vi "GetFullscreenDisplayModes.vi"(8 "No Error":errorcluster, 11 "DisplayID":T2) -> (0 "Error Out":errorcluster, 3 "Display Modes":T1[](array[typedef]))   [LabVIEW 2024, in "SDL3.lvlib" / "Video.lvlib"]
doc: "<B>Summary</B>\nGet a list of fullscreen display modes available on a display.\n\n<B>Remarks</B>\nThe display modes are sorted in this priority:\n\nw -> largest to smallest\nh -> largest to smallest\nbits per pixel -> more colors to fewer colors\npacked pixel layout -> largest to smallest\nrefresh rate -> highest to lowest\npixel density -> lowest to highest"
uses:
  Video.lvlib
  DisplayID--integer.ctl
  DisplayMode--cluster.ctl
  Pixels/PixelFormat--enum.ctl
  Dereference-DisplayMode.vi/d7f35e20-2a2c-4e03-b91a-a2fa7be3e3c2.vi
  Dereference-DisplayMode.vi/9072d7ce-49ca-4829-bd8f-b245b58a6c9d.vi
  Pixels/U32ToPixelFormatEnum.vi
  <vilib>/Utility/error.llb/Error Cluster From Error Code.vi
  Error/Error.lvlib
  Lib/SDL3-32.dll
  Stdinc/Stdinc.lvlib
  LV-Utilities/LV-Utilities.lvlib
  Pixels/Pixels.lvlib
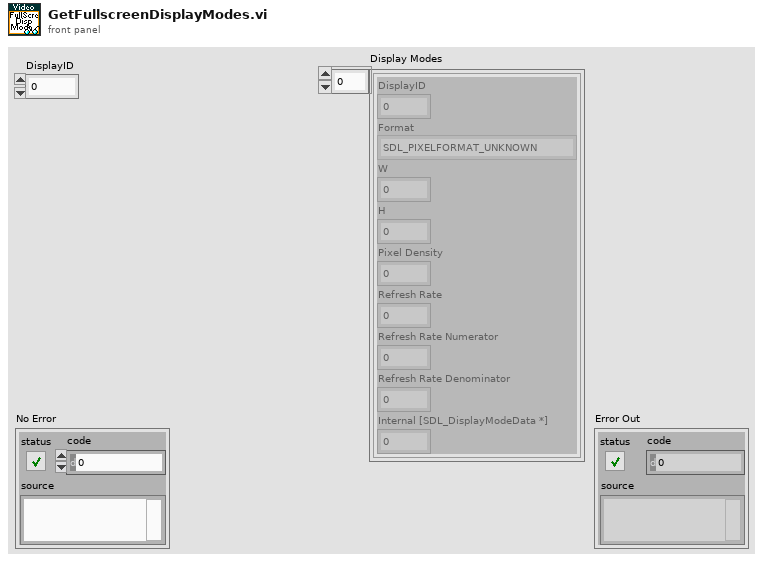
[diagram p1: front panel]
types:
  T1 = typedef "SDL3.lvlib/Video.lvlib/DisplayMode--cluster.ctl" = cluster{"DisplayID":T2, "Format":T3, "W":i32, "H":i32, "Pixel Density":sgl, "Refresh Rate":sgl, "Refresh Rate Numerator":i32, "Refresh Rate Denominator":i32, "Internal [SDL_DisplayModeData *]":i64}
  T2 = typedef "SDL3.lvlib/Video.lvlib/DisplayID--integer.ctl" = u32
  T3 = typedef "SDL3.lvlib/Pixels.lvlib/PixelFormat--enum.ctl" = enum32{"SDL_PIXELFORMAT_UNKNOWN", "SDL_PIXELFORMAT_INDEX1LSB", "SDL_PIXELFORMAT_INDEX1MSB", "SDL_PIXELFORMAT_INDEX2LSB", "SDL_PIXELFORMAT_INDEX2MSB", "SDL_PIXELFORMAT_INDEX4LSB", "SDL_PIXELFORMAT_INDEX4MSB", "SDL_PIXELFORMAT_INDEX8", "SDL_PIXELFORMAT_RGB332", "SDL_PIXELFORMAT_XRGB4444", "SDL_PIXELFORMAT_XBGR4444", "SDL_PIXELFORMAT_XRGB1555", "SDL_PIXELFORMAT_XBGR1555", "SDL_PIXELFORMAT_ARGB4444", "SDL_PIXELFORMAT_RGBA4444", "SDL_PIXELFORMAT_ABGR4444", "SDL_PIXELFORMAT_BGRA4444", "SDL_PIXELFORMAT_ARGB1555", "SDL_PIXELFORMAT_RGBA5551", "SDL_PIXELFORMAT_ABGR1555", "SDL_PIXELFORMAT_BGRA5551", "SDL_PIXELFORMAT_RGB565", "SDL_PIXELFORMAT_BGR565", "SDL_PIXELFORMAT_RGB24", "SDL_PIXELFORMAT_BGR24", "SDL_PIXELFORMAT_XRGB8888", "SDL_PIXELFORMAT_RGBX8888", "SDL_PIXELFORMAT_XBGR8888", "SDL_PIXELFORMAT_BGRX8888", "SDL_PIXELFORMAT_ARGB8888", "SDL_PIXELFORMAT_RGBA8888", "SDL_PIXELFORMAT_ABGR8888", "SDL_PIXELFORMAT_BGRA8888", "SDL_PIXELFORMAT_XRGB2101010", "SDL_PIXELFORMAT_XBGR2101010", "SDL_PIXELFORMAT_ARGB2101010", "SDL_PIXELFORMAT_ABGR2101010", "SDL_PIXELFORMAT_RGB48", "SDL_PIXELFORMAT_BGR48", "SDL_PIXELFORMAT_RGBA64", "SDL_PIXELFORMAT_ARGB64", "SDL_PIXELFORMAT_BGRA64", "SDL_PIXELFORMAT_ABGR64", "SDL_PIXELFORMAT_RGB48_FLOAT", "SDL_PIXELFORMAT_BGR48_FLOAT", "SDL_PIXELFORMAT_RGBA64_FLOAT", "SDL_PIXELFORMAT_ARGB64_FLOAT", "SDL_PIXELFORMAT_BGRA64_FLOAT", "SDL_PIXELFORMAT_ABGR64_FLOAT", "SDL_PIXELFORMAT_RGB96_FLOAT", "SDL_PIXELFORMAT_BGR96_FLOAT", "SDL_PIXELFORMAT_RGBA128_FLOAT", "SDL_PIXELFORMAT_ARGB128_FLOAT", "SDL_PIXELFORMAT_BGRA128_FLOAT", "SDL_PIXELFORMAT_ABGR128_FLOAT", "SDL_PIXELFORMAT_YV12", "SDL_PIXELFORMAT_IYUV", "SDL_PIXELFORMAT_YUY2", "SDL_PIXELFORMAT_UYVY", "SDL_PIXELFORMAT_YVYU", "SDL_PIXELFORMAT_NV12", "SDL_PIXELFORMAT_NV21", "SDL_PIXELFORMAT_P010", "SDL_PIXELFORMAT_EXTERNAL_OES"}
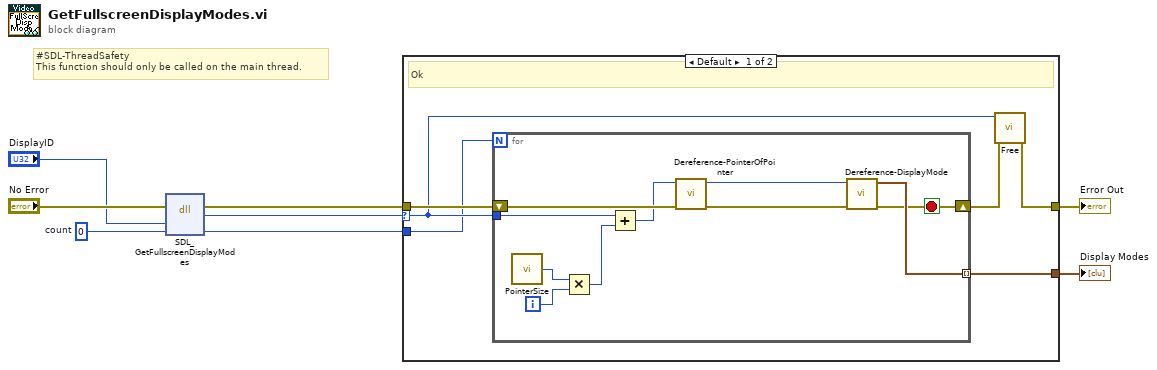
[diagram p0: block diagram]
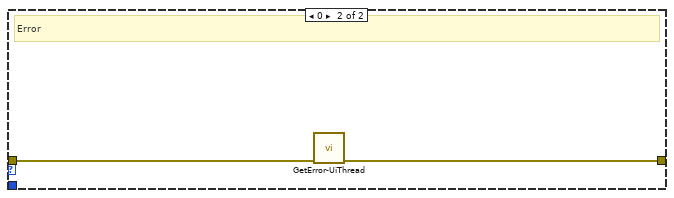
[diagram p2: hidden frame]
diagram:
  w2 = 0  # count
  # "#SDL-ThreadSafety\nThis function should only be called on the main thread."
  n1 = dll-call lib="C:/Users/Thomas/Documents/Projects/LV-SDL3/Lib/SDL3-*.*" fn="SDL_GetFullscreenDisplayModes"(error in="No Error", "displayID"="DisplayID", "count"=w2) -> (error out=w6:errorcluster, "return type"=w4:i64, "count"=w1:i32)  [unwired: 3 in, 1 out]
  n2 = case shown="Default" w4 {
    selector: w4 -> [w12 _]
    tunnel: w6 -> [w13 w26]
    tunnel: [w10 w25] -> w5
    tunnel: [w14 _] -> w3
    tunnel: w1 -> [w9 _]
    frame Default {
      # "Ok"
      n3 = for {
        N: w9 -> [_]
        tunnel: w12 -> [w24]
        tunnel: [w23] -> w14 mode=indexing
        shift-right: [w15] -> w11
        shift-left: w13 -> [w20]
        i -> [w22]
        stop <- w15 stop-if-true
        n4 = call "PointerSize.vi"() -> ("Pointer Size [Byte]"=w19:i32)
        n5 = Multiply(x=w19, y=w22) -> (x*y=w21:i32)
        n6 = Add(x=w24, y=w21) -> (x+y=w18:i64)
        n7 = call "Dereference-PointerOfPointer.vi"("No Error"=w20, "Ptr of Ptr [void **]"=w18) -> ("error out"=w16:errorcluster, "Ptr [void *]"=w17:i64)  [unwired: 8 in]
        n8 = call "Dereference-DisplayMode.vi"("error in (no error)"=w16, "[SDL_DisplayMode*]"=w17) -> ("error out"=w15:errorcluster, "Display Mode"=w23:T1)  [unwired: 8 in]
      }
      n9 = call "Free.vi"("No Error"=w11, "Mem [void *]"=w12) -> ("Error Out"=w10:errorcluster)  [unwired: 9 in]
    }
    frame 0 {
      # "Error"
      n10 = call "GetError-UiThread.vi"("No Error"=w26) -> ("error out"=w25:errorcluster)  [unwired: 10 in]
    }
  }
  "Error Out" <- w5
  "Display Modes" <- w3
